vi "Determine ConPane Pattern.vi"(1 "Connector Panes":u16(ring)=3) -> (0 "Pattern Value":u32)   [LabVIEW 2017]
doc: "Select a Connector Pane pattern in the ring and run the VI to find out the pattern number."
panel:
  # "Select a Connector Pane pattern in the ring and run the VI to find out the pattern number."
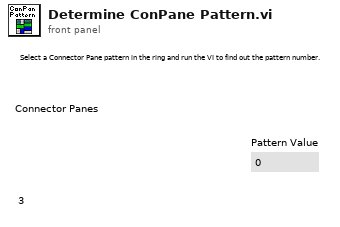
[diagram p1: front panel]
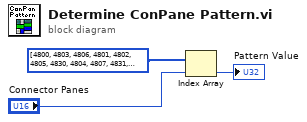
[diagram p0: block diagram]
diagram:
  n1 = Index Array(array=u32[] [4800, 4803, 4806, 4801, 4802, 4805, 4830, 4804, 4807, 4831, 4832, 4810, 4808, 4809, 4811, 4812, 4816, 4823, 4824, 4817, 4818, 4825, 4819, 4813, 4820, 4826, 4821, 4827, 4828, 4822, 4814, 4829, 4815, 4833, 4834, 4835], index="Connector Panes") -> (element=→"Pattern Value":u32)
